vi "Exit In Place Element DVR.vi"(0 "Diagram in":refnum<vi>, 5 "Data Value":refnum<vi>, 7 "Outputs":refnum<vi>[](array[refnum]), 11 "error in (no error)":errorcluster) -> (4 "Diagram out":refnum<vi>, 6 "DVR":refnum<vi>, 8 "Outputs":refnum<vi>[](array[refnum]), 10 "DVR Error":refnum<vi>, 15 "error out":errorcluster)   [LabVIEW 2015, in "Scripting.lvlib"]
doc: "Exits the In Place Element Structure that owns <B>Diagram in</B>, supplying the structure's owning diagram at <B>Diagram out</B>.\n\n<B>Data Value</B> is the terminal to wire to the Write Data Value Reference node's data value terminal.\n\n<B>DVR</B> is the data value reference output terminal of the Write Data Value Reference node.\n\n<B>DVR Error</B> is the error output terminal of the Write Data Value Reference node."
uses:
  Scripting.lvlib
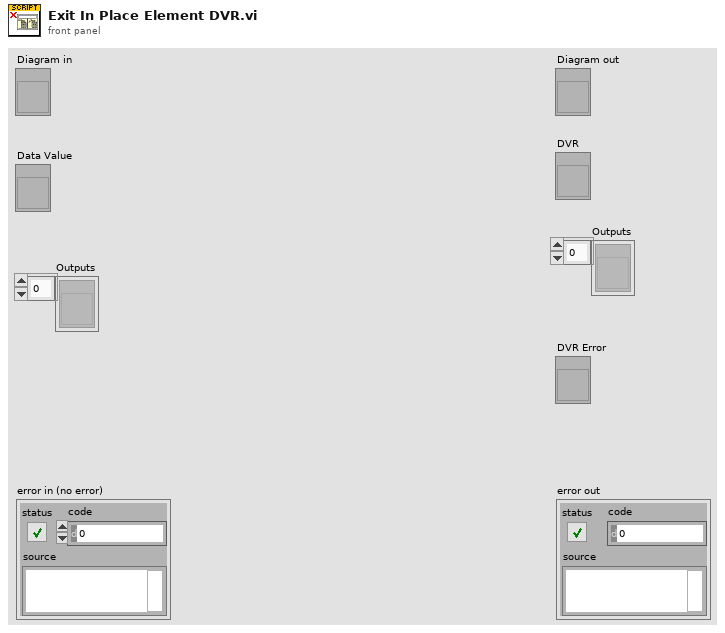
[diagram p1: front panel]
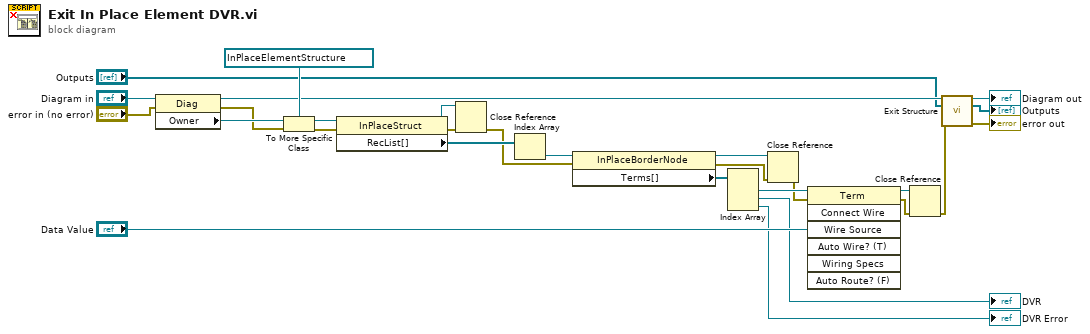
[diagram p0: block diagram]
diagram:
  n1 = property class="Diag"(reference="Diagram in", error in="error in (no error)") -> (reference out=w11:refnum<vi>, error out=w13:errorcluster, "Owner"=w26:refnum<vi>)
  n2 = To More Specific Class(target class=refnum<vi> refnum ("reference"), reference=w26, error in=w13) -> (specific class reference=w21:refnum<vi>, error out=w24:errorcluster)
  n3 = property class="InPlaceStruct"(reference=w21, error in=w24) -> (reference out=w5:refnum<vi>, error out=w25:errorcluster, "RecList[]"=w22:refnum<vi>[])
  n4 = Close Reference(reference=w5, error in (no error)=w25) -> (error out=w6:errorcluster)
  n5 = Index Array(array=w22) -> (element=w23:refnum<vi>)  [unwired: 1 in]
  n6 = property class="InPlaceBorderNode"(reference=w23, error in=w6) -> (reference out=w3:refnum<vi>, error out=w28:errorcluster, "Terms[]"=w19:refnum<vi>[])
  n7 = Index Array(array=w19) -> (element #1=w27:refnum<vi>, element #2=→"DVR":refnum<vi>, element #3=→"DVR Error":refnum<vi>)  [unwired: 3 in]
  n8 = Close Reference(reference=w3, error in (no error)=w28) -> (error out=w4:errorcluster)
  n9 = invoke class="Term" method="Connect Wire"(reference=w27, error in=w4, "Wire Source"="Data Value") -> (reference out=w1:refnum<vi>, error out=w12:errorcluster)  [unwired: 4 in, 5 out]
  n10 = Close Reference(reference=w1, error in (no error)=w12) -> (error out=w2:errorcluster)
  n11 = call "Exit Structure.vi"("Diagram in"=w11, "Outputs"="Outputs", "error in (no error)"=w2) -> ("Diagram out"=→"Diagram out":refnum<vi>, "Outputs"=→"Outputs":refnum<vi>[], "error out"=→"error out":errorcluster)  [unwired: 10 in]
